vi "Create Detrough Envelope Waveform.vi"(0 "Reference Waveform":T3 {"Runtime Scaling" format="%#_6p"; "Sample Rate" format="%#_6p"; "Burst Length (s)" format="%#_6p"; "PAPR (dB)" format="%.2f"; "Signal Bandwidth (Hz)" format="%#_6p"}, 5 "Detrough Configuration":T1={"Type"=enum."Exponential", "Minimum Voltage (V)"=1.5, "Maximum Voltage (V)"=3.5, "Exponent"=1.2000000476837158}, 11 "error in (no error)":errorcluster) -> (4 "Detrough Envelope Waveform":T3 {"Runtime Scaling" format="%#_6p"; "Sample Rate" format="%#_6p"; "Burst Length (s)" format="%#_6p"; "PAPR (dB)" format="%.2f"; "Signal Bandwidth (Hz)" format="%#_6p"}, 15 "error out":errorcluster)   [LabVIEW 2016, in "Envelope Tracking.lvlib"]
uses:
  Envelope Tracking.lvlib
  Common/Waveform.ctl
  Typedefs/Detrough Configuration.ctl
  Typedefs/Detrough Type.ctl
  Common/Common.lvlib
  <vilib>/addons/ET/niETUtil/niETUtil.lvlib
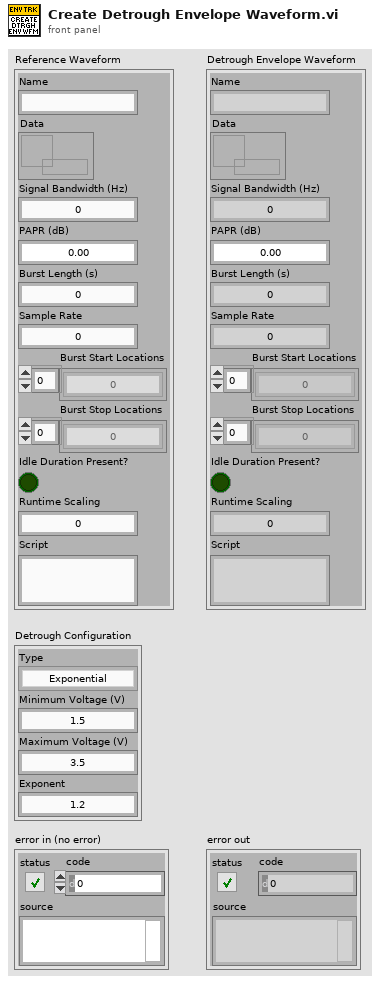
[diagram p1: front panel]
types:
  T1 = typedef "Envelope Tracking.lvlib/Detrough Configuration.ctl" = cluster{"Type":T2, "Minimum Voltage (V)":dbl, "Maximum Voltage (V)":dbl, "Exponent":dbl}
  T2 = typedef "Envelope Tracking.lvlib/Detrough Type.ctl" = enum16{"Exponential", "Cosine", "Power"}
  T3 = typedef "Common.lvlib/Waveform.ctl" = cluster{"Name":string, "Data":refnum<data-value>, "Signal Bandwidth (Hz)":dbl, "PAPR (dB)":dbl, "Burst Length (s)":dbl, "Sample Rate":dbl, "Burst Start Locations":i32[], "Burst Stop Locations":i32[], "Idle Duration Present?":bool, "Runtime Scaling":dbl, "Script":string}
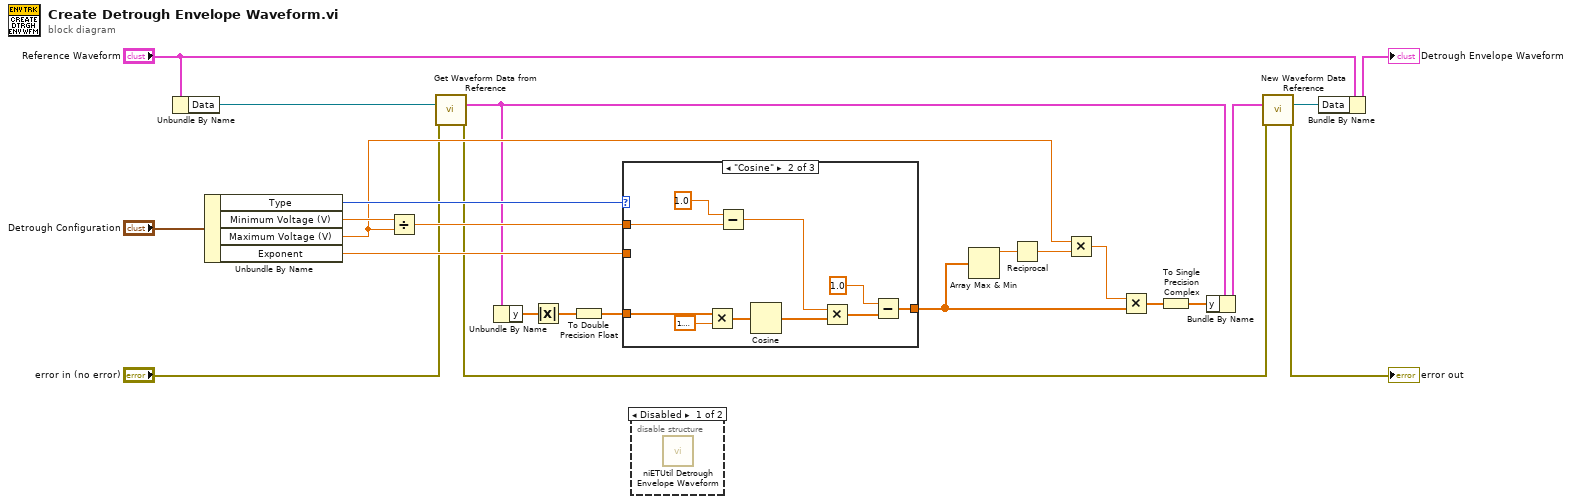
[diagram p0: block diagram]
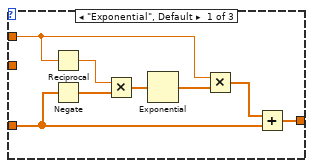
[diagram p2: hidden frame]
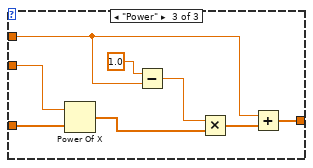
[diagram p3: hidden frame]
diagram:
  n1 = Unbundle By Name("Reference Waveform") -> ("Data"=w15:refnum<data-value>)
  n2 = Unbundle By Name("Detrough Configuration") -> ("Type"=w19:T2, "Minimum Voltage (V)"=w18:dbl, "Maximum Voltage (V)"=w17:dbl, "Exponent"=w16:dbl)
  n3 = Divide(x=w18, y=w17) -> (x/y=w21:dbl)
  n4 = call "Get Waveform Data from Reference.vi"("Waveform Data Reference"=w15, "error in (no error)"="error in (no error)") -> ("Waveform Data"=w8:cluster{"t0":dbl, "dt":dbl, "y":csg[]}, "error out"=w5:errorcluster)  [unwired: 12 in]
  n5 = Unbundle By Name(w8) -> ("y"=w14:csg[])
  n6 = Absolute Value(x=w14) -> (abs(x)=w11:sgl[])
  n7 = To Double Precision Float(number=w11) -> (double precision float=w10:dbl[])
  n8 = case shown="\"Cosine\"" w19 {
    tunnel: w10 -> [w26 w42 w50]
    tunnel: w21 -> [w28 w34 w44]
    tunnel: [w25 w37 w46] -> w13
    tunnel: w16 -> [_ _ w49]
    frame "Exponential", Default {
      n9 = Reciprocal(x=w28) -> (1/x=w30:dbl)
      n10 = Negate(x=w26) -> (-x=w32:dbl[])
      n11 = Multiply(x=w30, y=w32) -> (x*y=w31:dbl[])
      n12 = Exponential(1:w31) -> (0:w29:dbl[])
      n13 = Multiply(x=w28, y=w29) -> (x*y=w27:dbl[])
      n14 = Add(x=w27, y=w26) -> (x+y=w25:dbl[])
    }
    frame "Cosine" {
      n15 = Multiply(x=w42, y=1.5707963267948966) -> (x*y=w41:dbl[])
      n16 = Subtract(x=1.0, y=w34) -> (x-y=w33:dbl)
      n17 = Cosine(x=w41) -> (cos(x)=w40:dbl[])
      n18 = Multiply(x=w33, y=w40) -> (x*y=w38:dbl[])
      n19 = Subtract(x=1.0, y=w38) -> (x-y=w37:dbl[])
    }
    frame "Power" {
      n20 = Power Of X(1:w50, 2:w49) -> (0:w48:dbl[])
      n21 = Subtract(x=1.0, y=w44) -> (x-y=w43:dbl)
      n22 = Multiply(x=w43, y=w48) -> (x*y=w47:dbl[])
      n23 = Add(x=w44, y=w47) -> (x+y=w46:dbl[])
    }
  }
  n24 = disable-structure shown="Disabled" {
    frame Disabled {
      n25 = call <vilib>:"niETUtil Detrough Envelope Waveform.vi"() -> ()  [unwired: 12 in, 4 out]
    }
    frame Enabled {
    }
  }
  n26 = Array Max & Min(array=w13) -> (max value=w23:dbl)  [unwired: 3 out]
  n27 = Reciprocal(x=w23) -> (1/x=w22:dbl)
  n28 = Multiply(x=w17, y=w22) -> (x*y=w20:dbl)
  n29 = Multiply(x=w20, y=w13) -> (x*y=w9:dbl[])
  n30 = To Single Precision Complex(1:w9) -> (0:w7:csg[])
  n31 = Bundle By Name(cluster=w8, "y"=w7) -> (w6:cluster{"t0":dbl, "dt":dbl, "y":csg[]})
  n32 = call "New Waveform Data Reference.vi"("Waveform Data"=w6, "error in (no error)"=w5) -> ("Waveform Data Reference"=w3:refnum<data-value>, "error out"=→"error out":errorcluster)  [unwired: 12 in]
  n33 = Bundle By Name(cluster="Reference Waveform", "Data"=w3) -> (→"Detrough Envelope Waveform":T3)
